vi "scale raw ESR.vi"(8 "error in (no error)":errorcluster, 10 "ESR scaling":T8[](array[typedef]), 11 "Processing loop variables":T1 {"CurrInverter"."last updated" format="%<%H:%M\n%d/%m/%Y>T"; "CurrInverter"."set flag" items=["False", "True"]}) -> (0 "error out":errorcluster, 3 "Processing loop variables out":T1 {"CurrInverter"."last updated" format="%<%H:%M\n%d/%m/%Y>T"; "CurrInverter"."set flag" items=["False", "True"]})   [LabVIEW 2019, in "Main.lvclass"]
doc: "Developed by Kevin Thompson\nkevin@thompsonengineering.net\n\nCopyright 2020\nThompson Engineering, LLC"
uses:
  Main.lvclass
  DataTypes/Processing loop variables--cluster.ctl
  DataTypes/averaging variables.ctl
  DataTypes/ESR alarm variables.ctl
  Common/DataTypes/Inverter database record v2--cluster.ctl
  Common/DataTypes/inverter info v2--cluster.ctl
  Common/DataTypes/inverter gain range--cluster.ctl
  Common/DataTypes/inverter offset range--cluster.ctl
  DataTypes/ESR scaling--cluster.ctl
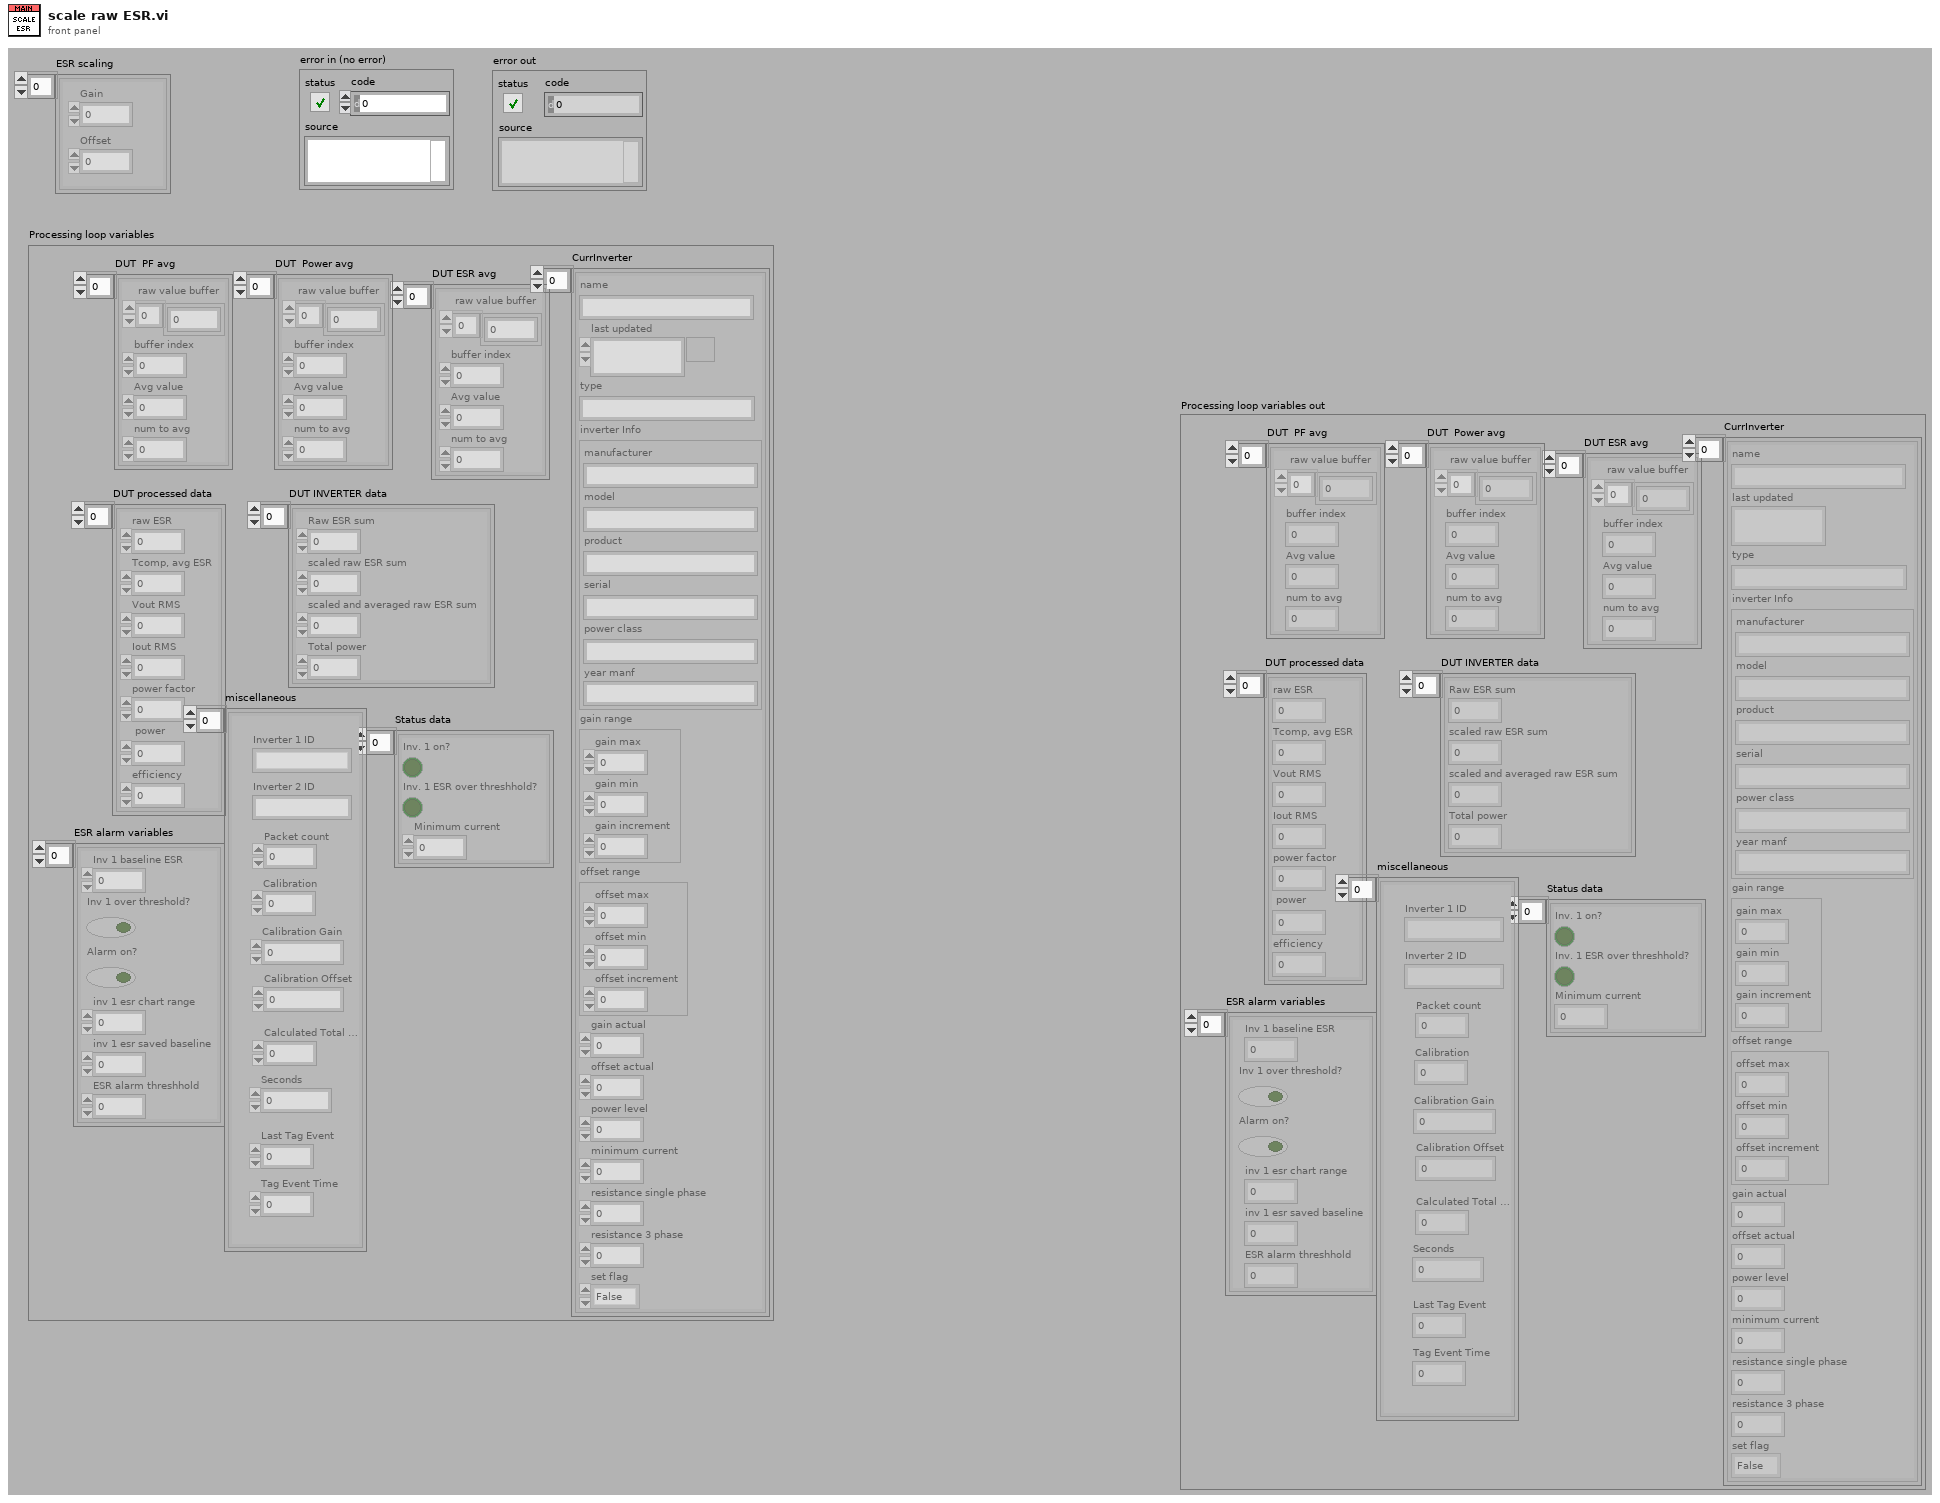
[diagram p1: front panel]
types:
  T1 = typedef "Main.lvclass/Processing loop variables--cluster.ctl" = cluster{"DUT ESR avg":T2[], "DUT  PF avg":T2[], "DUT  Power avg ":T2[], "DUT processed data":cluster{"raw ESR":dbl, "Tcomp, avg ESR":dbl, "Vout RMS":dbl, "Iout RMS":dbl, "power factor":dbl, "power":dbl, "efficiency":dbl}[], "ESR alarm variables":T3[], "Status data":cluster{"Inv. 1 on?":bool, "Inv. 1 ESR over threshhold?":bool, "Minimum current":dbl}[], "CurrInverter":T4[], "miscellaneous":cluster{"Inverter 1 ID":string, "Inverter 2 ID":string, "Packet count":u32, "Calibration":dbl, "Calibration Gain":dbl, "Calibration Offset":dbl, "Calculated Total Power":dbl, "Seconds":dbl, "Last Tag Event":dbl, "Tag Event Time":dbl}[], "DUT INVERTER data":cluster{"Raw ESR sum":dbl, "scaled raw ESR sum":dbl, "scaled and averaged raw ESR sum":dbl, "Total power":dbl}[]}
  T2 = typedef "Main.lvclass/averaging variables.ctl" = cluster{"raw value buffer":dbl[], "buffer index":i32, "Avg value":dbl, "num to avg":i32}
  T3 = typedef "Main.lvclass/ESR alarm variables.ctl" = cluster{"Inv 1 baseline ESR":dbl, "Inv 1 over threshold?":bool, "Alarm on?":bool, "inv 1 esr chart range":dbl, "inv 1 esr saved baseline":dbl, "ESR alarm threshhold":dbl}
  T4 = typedef "Inverter database record v2--cluster.ctl" = cluster{"name":string, "last updated":timestamp, "type":string, "inverter Info":T5, "gain range":T6, "offset range":T7, "gain actual":dbl, "offset actual":dbl, "power level":dbl, "minimum current":dbl, "resistance single phase":dbl, "resistance 3 phase":dbl, "set flag":u16}
  T5 = typedef "inverter info v2--cluster.ctl" = cluster{"manufacturer":string, "model":string, "product":string, "serial":string, "power class":string, "year manf":string}
  T6 = typedef "inverter gain range--cluster.ctl" = cluster{"gain max":dbl, "gain min":dbl, "gain increment":dbl}
  T7 = typedef "inverter offset range--cluster.ctl" = cluster{"offset max":dbl, "offset min":dbl, "offset increment":dbl}
  T8 = typedef "Main.lvclass/ESR scaling--cluster.ctl" = cluster{"Gain":dbl, "Offset":dbl}
  T9 = cluster{"Raw ESR sum":dbl, "scaled raw ESR sum":dbl, "scaled and averaged raw ESR sum":dbl, "Total power":dbl}[]
  T10 = cluster{"raw ESR":dbl, "Tcomp, avg ESR":dbl, "Vout RMS":dbl, "Iout RMS":dbl, "power factor":dbl, "power":dbl, "efficiency":dbl}[]
  T11 = cluster{"Raw ESR sum":dbl, "scaled raw ESR sum":dbl, "scaled and averaged raw ESR sum":dbl, "Total power":dbl}
  T12 = cluster{"raw ESR":dbl, "Tcomp, avg ESR":dbl, "Vout RMS":dbl, "Iout RMS":dbl, "power factor":dbl, "power":dbl, "efficiency":dbl}
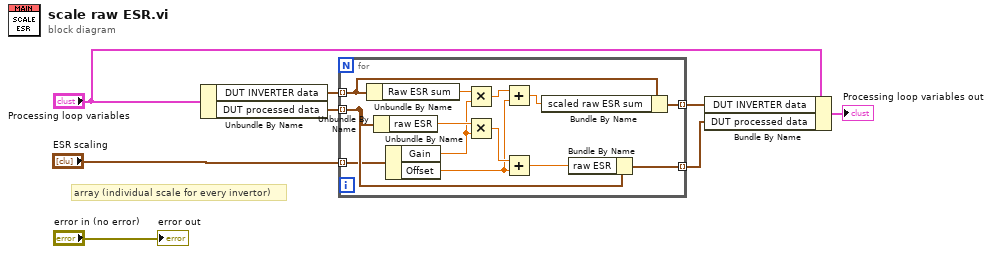
[diagram p0: block diagram]
diagram:
  # "array (individual scale for every invertor)"
  n1 = Unbundle By Name("Processing loop variables") -> ("DUT INVERTER data"=w3:T9, "DUT processed data"=w7:T10)
  n2 = for {
    tunnel: w7 -> [w21] mode=indexing
    tunnel: [w19] -> w4 mode=indexing
    tunnel: w3 -> [w14] mode=indexing
    tunnel: [w12] -> w2 mode=indexing
    tunnel: "ESR scaling" -> [w11] mode=indexing
    n3 = Unbundle By Name(w14) -> ("Raw ESR sum"=w18:dbl)
    n4 = Unbundle By Name(w21) -> ("raw ESR"=w16:dbl)
    n5 = Unbundle By Name(w11) -> ("Gain"=w10:dbl, "Offset"=w9:dbl)
    n6 = Multiply(x=w18, y=w10) -> (x*y=w20:dbl)
    n7 = Multiply(x=w16, y=w10) -> (x*y=w17:dbl)
    n8 = Add(x=w20, y=w9) -> (x+y=w13:dbl)
    n9 = Add(x=w17, y=w9) -> (x+y=w15:dbl)
    n10 = Bundle By Name(cluster=w14, "scaled raw ESR sum"=w13) -> (w12:T11)
    n11 = Bundle By Name(cluster=w21, "raw ESR"=w15) -> (w19:T12)
  }
  n12 = Bundle By Name(cluster="Processing loop variables", "DUT INVERTER data"=w2, "DUT processed data"=w4) -> (→"Processing loop variables out":T1)
  "error out" <- "error in (no error)"
